vi "Check Rotation Coordinates.vi"(4 "Wall Positions":T4[](array[typedef]), 6 "GameBoard Size":T4, 8 "Error In":errorcluster caption="Entrée d'erreur", 9 "New Rotation State":T1, 10 "Rotated Coordinates":T4[](array[typedef]), 11 "Piece description":T2) -> (0 "Error Out":errorcluster caption="Sortie d'erreur", 3 "Piece description Out":T2)   [LabVIEW 2017]
uses:
  Controls/Coordinates.ctl
  Controls/Piece Description.ctl
  Controls/Pieces Geometry Names.ctl
  Controls/Rotation State.ctl
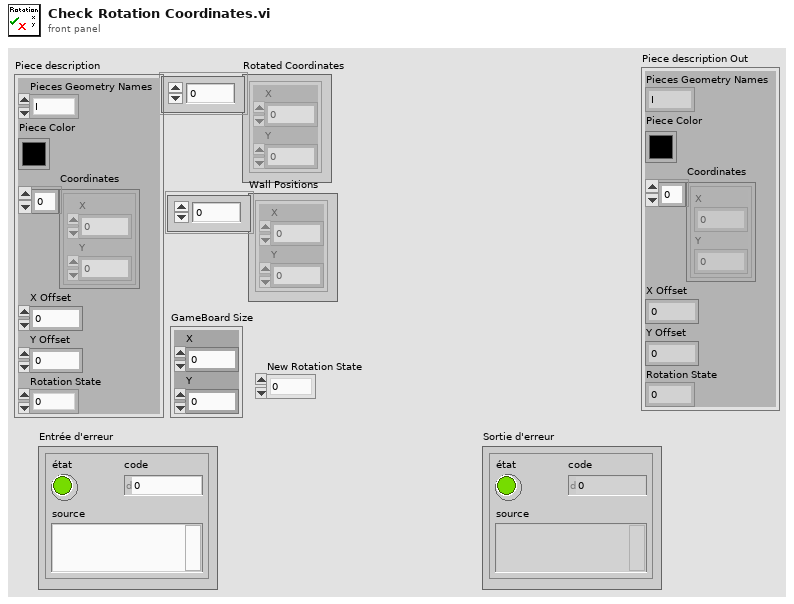
[diagram p1: front panel]
types:
  T1 = typedef "Rotation State.ctl" = enum16{"0", "90", "180", "270"}
  T2 = typedef "Piece Description.ctl" = cluster{"Pieces Geometry Names":T3, "Piece Color":u32, "Coordinates":T4[], "X Offset":i32, "Y Offset":i32, "Rotation State":T1}
  T3 = typedef "Pieces Geometry Names.ctl" = enum16{"I", "O", "T", "L", "J", "Z", "S"}
  T4 = typedef "Coordinates.ctl" = cluster{"X":i32, "Y":i32}
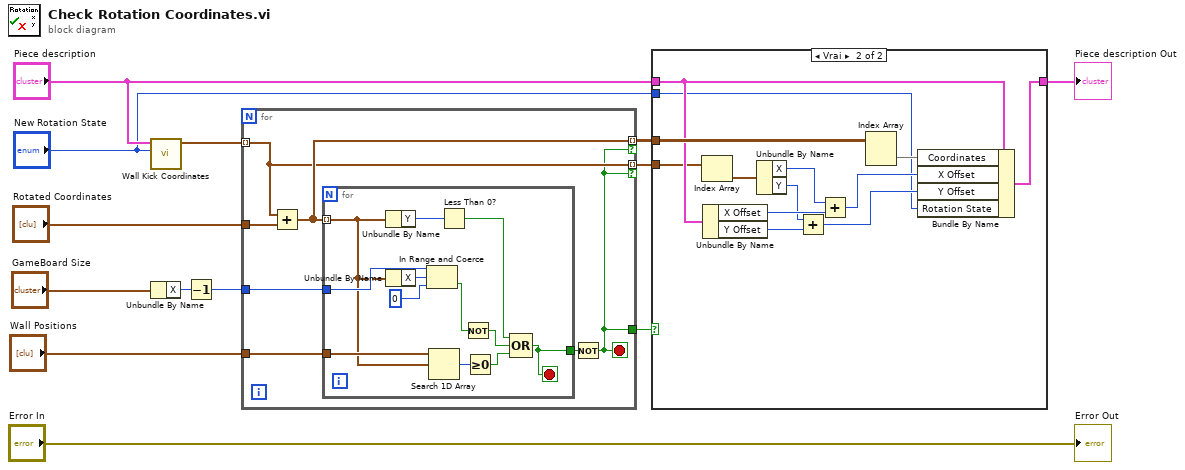
[diagram p0: block diagram]
diagram:
  n1 = call "Wall Kick Coordinates.vi"("New Rotation State"="New Rotation State", "Piece description"="Piece description") -> ("Test Coordinates"=w5:T4[])  [unwired: 8 in, 1 out]
  n2 = Unbundle By Name("GameBoard Size") -> ("X"=w10:i32)
  n3 = Decrement(x=w10) -> (x-1=w11:i32)
  n4 = for {
    tunnel: "Rotated Coordinates" -> [w20]
    tunnel: "Wall Positions" -> [w19]
    tunnel: w11 -> [w18]
    tunnel: w5 -> [w15] mode=indexing
    tunnel: [w14] -> w4
    tunnel: [w16] -> w3 mode=indexing if=w14
    tunnel: [w15] -> w2 mode=indexing if=w14
    stop <- w14 stop-if-true
    n5 = Add(x=w15, y=w20) -> (x+y=w16:T4[])
    n6 = for {
      tunnel: w18 -> [w31]
      tunnel: w16 -> [w21] mode=indexing
      tunnel: w19 -> [w27]
      tunnel: [w24] -> w17
      stop <- w24 stop-if-true
      n7 = Unbundle By Name(w21) -> ("Y"=w23:i32)
      n8 = Unbundle By Name(w21) -> ("X"=w32:i32)
      n9 = In Range and Coerce(upper limit=w31, x=w32, lower limit=0 ("limite inférieure")) -> (In Range?=w29:bool)  [unwired: 1 out]
      n10 = Search 1D Array(1D array=w27, element=w21) -> (index of element=w28:i32)  [unwired: 1 in]
      n11 = Less Than 0?(x=w23) -> (x < 0?=w22:bool)
      n12 = Not(x=w29) -> (.not. x?=w25:bool)
      n13 = Greater Or Equal To 0?(x=w28) -> (x >= 0?=w26:bool)
      n14 = Compound Arithmetic op=OR ("Opérateur arithmétique")(w22, w25, w26) -> (w24:bool)
    }
    n15 = Not(x=w17) -> (.not. x?=w14:bool)
  }
  n16 = case shown="Vrai" w4 {
    tunnel: "Piece description" -> [w33 w43]
    tunnel: [w33 w46] -> w7
    tunnel: w3 -> [_ w45]
    tunnel: w2 -> [_ w42]
    tunnel: "New Rotation State" -> [_ w34]
    frame False {
    }
    frame True {
      n17 = Index Array(array=w42) -> (element=w41:T4)  [unwired: 1 in]
      n18 = Unbundle By Name(w43) -> ("X Offset"=w39:i32, "Y Offset"=w37:i32)
      n19 = Unbundle By Name(w41) -> ("X"=w40:i32, "Y"=w36:i32)
      n20 = Add(x=w36, y=w37) -> (x+y=w35:i32)
      n21 = Add(x=w40, y=w39) -> (x+y=w38:i32)
      n22 = Index Array(array=w45) -> (element=w44:T4[])  [unwired: 2 in]
      n23 = Bundle By Name(cluster=w43, "Coordinates"=w44, "X Offset"=w38, "Y Offset"=w35, "Rotation State"=w34) -> (w46:T2)
    }
  }
  "Piece description Out" <- w7
  "Error Out" <- "Error In"
